vi "LvJDS2900SignalGeneratorApp.vi"() -> ()   [LabVIEW 2014]
uses:
  <vilib>/Utility/sysdir.llb/System Directory Type.ctl
  <vilib>/Utility/miscctls.llb/LVPointTypeDef.ctl
  <vilib>/Utility/error.llb/DialogType.ctl
  <vilib>/Instr/_visa.llb/VISA Configure Serial Port (Serial Instr).vi
  <vilib>/regexp/Match Regular Expression.xnode
panel:
  out "title":string="LvJDS2900SignalGeneratorApp"
  in  "Phase":dbl min=0.0 max=359.9 step=0.1 format="%0.1f"
  in  "Output 2":bool caption="Output"
  in  "Output 1":bool caption="Output"
  in  "Duty 2":dbl=50.0 caption="Duty" min=0.1 max=99.9 format="%04.1f"
  in  "Offset 2":dbl caption="Offset" min=-9.9 max=9.9 format="%04.2f"
  in  "Amplitude 2":dbl=5.0 caption="Amplitude" min=0.002 max=20.0 format="%06.3f"
  in  "WaveType 2":u16(ring) caption="WaveType" items=["Sine", "Square", "Pulse", "Triangle", "PartialSine", "CMOS", "DC"]
  in  "Frequency 2":dbl=1.0 caption="Frequency" min=1.0 max=60000000.0 format="%010.2f"
  in  "Duty 1":dbl=50.0 caption="Duty" min=0.1 max=99.9 format="%04.1f"
  in  "Offset 1":dbl caption="Offset" min=-9.99 max=9.99 format="%04.2f"
  in  "Amplitude 1":dbl=5.0 caption="Amplitude" min=0.002 max=20.0 format="%06.3f"
  in  "WaveType 1":u16(ring) caption="WaveType" items=["Sine", "Square", "Pulse", "Triangle", "PartialSine", "CMOS", "DC"]
  in  "Frequency 1":dbl=1.0 caption="Frequency" min=1.0 max=60000000.0 format="%010.2f"
  in  "VISA rscname":refnum<visa-resource-name>="COM3" caption="Port"
  in  "Btn Update":bool
  out "ModelName":string
  out "SerialNumber":string
  # "Unofficial JDS-2900 LvApp"
  # "Require NI-VISA\n\nConnect to PC via USB"
  # "As soon as the data is changed it will be sent to the device."
  # "CH1"
  # "CH2"
  # "Hz"
  # "V"
  # "V"
  # "%"
  # "Hz"
  # "V"
  # "V"
  # "%"
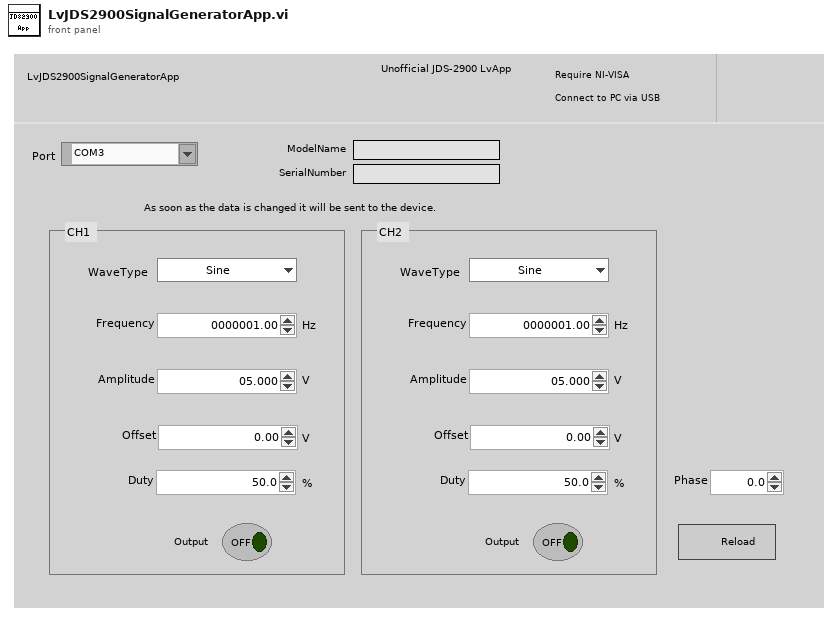
[diagram p1: front panel]
types:
  T1 = typedef "System Directory Type.ctl" = i32
  T2 = typedef "LVPointTypeDef.ctl" = cluster{"Horizontal":i16, "Vertical":i16}
  T3 = cluster{bool, "include Ctrl key?":bool, string}[]
  T4 = typedef "DialogType.ctl" = u16
  T5 = enum32{"invalid app kind", "Development System", "Run Time System", "Student Edition", "Embedded LabVIEW", "Evaluation", "Custom"}
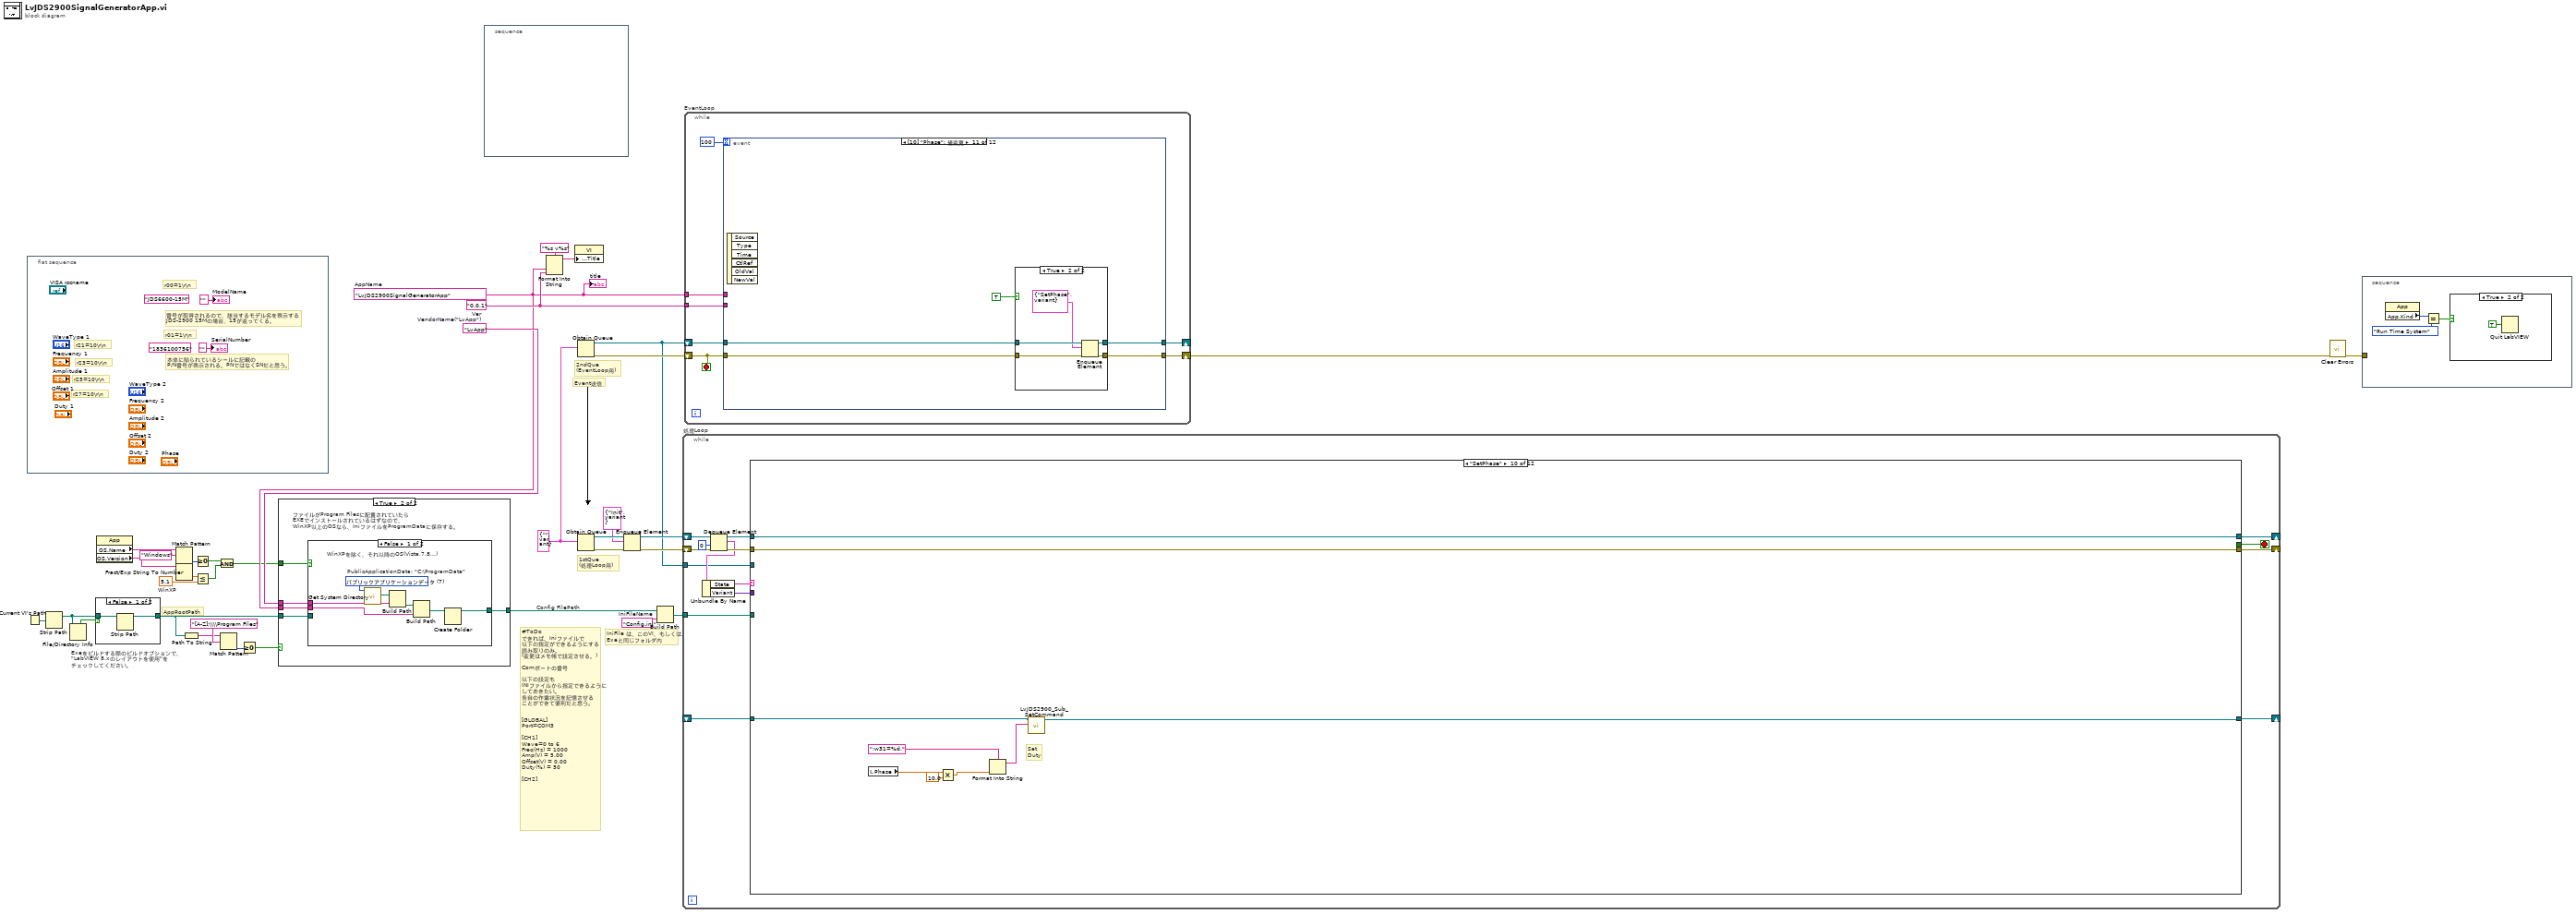
[diagram p0: block diagram]
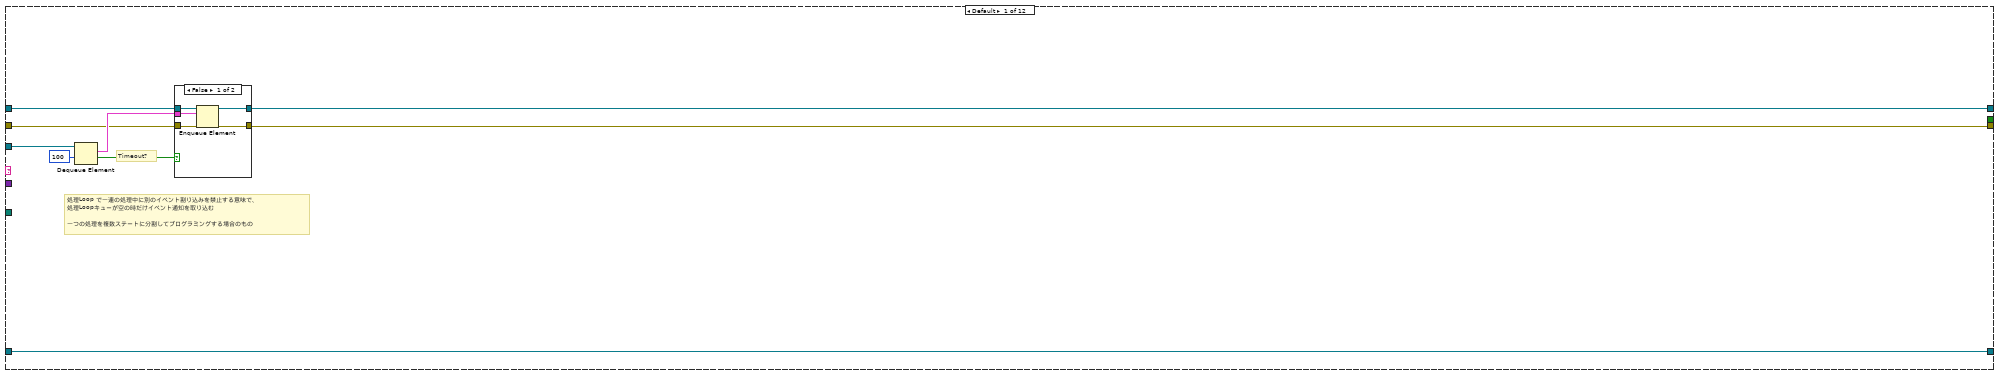
[diagram p6: hidden frame]
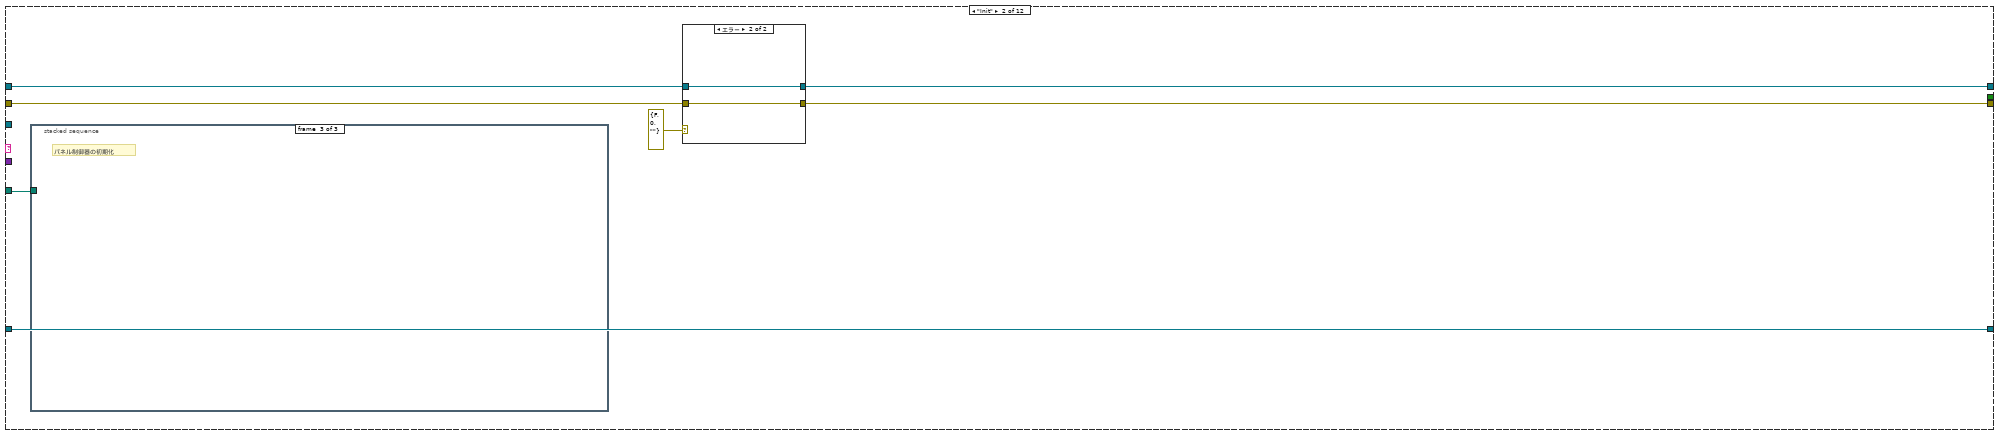
[diagram p8: hidden frame]
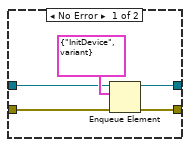
[diagram p9: hidden frame]
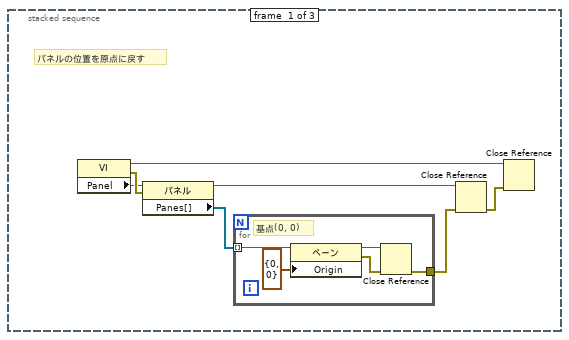
[diagram p10: hidden frame]
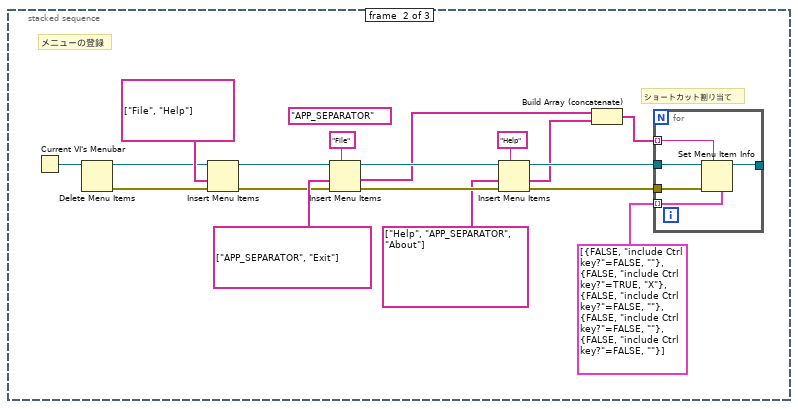
[diagram p11: hidden frame]
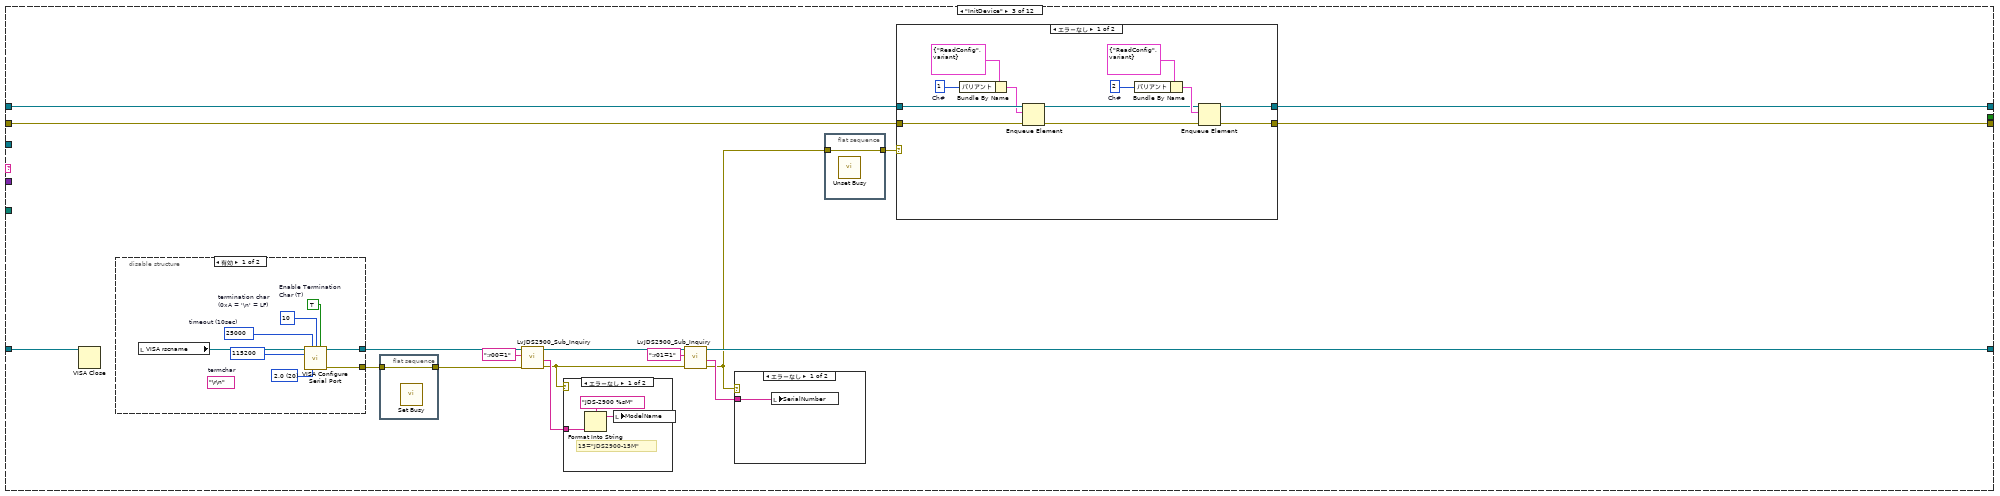
[diagram p12: hidden frame]
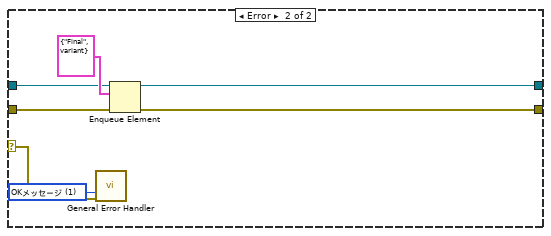
[diagram p15: hidden frame]
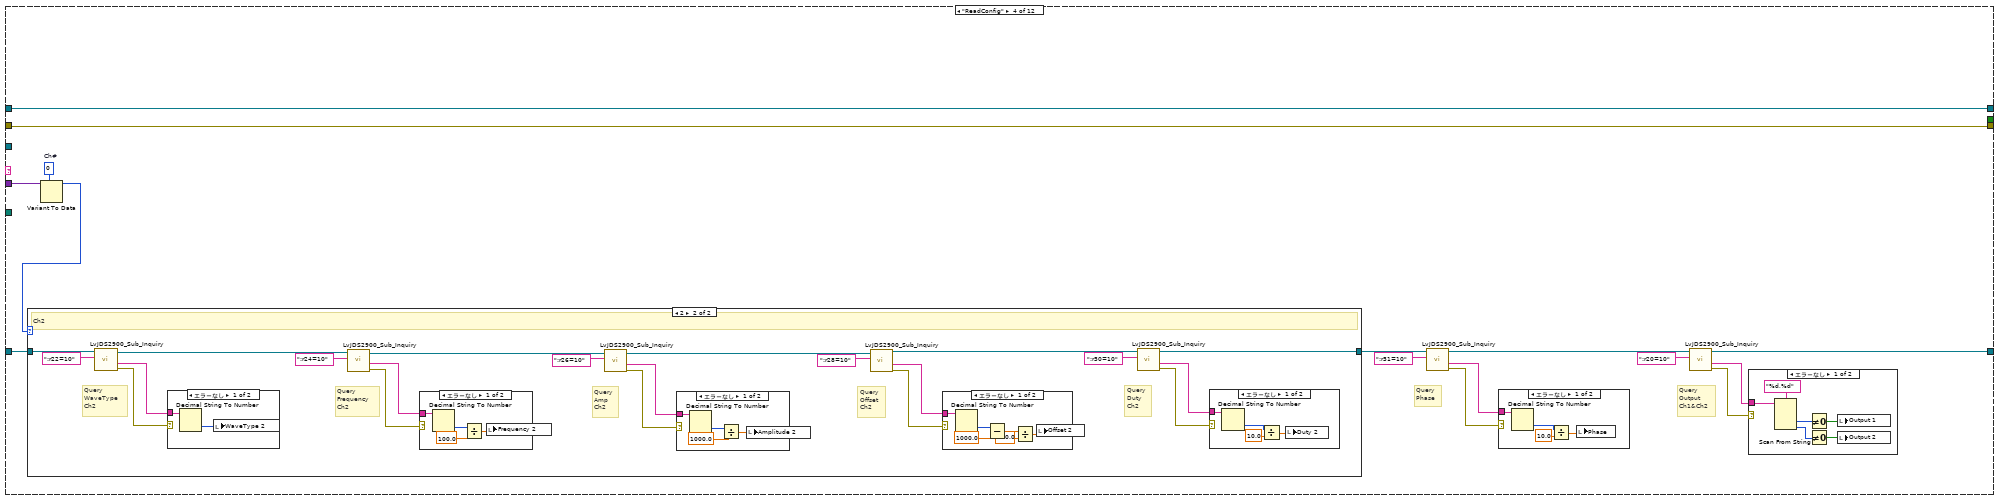
[diagram p17: hidden frame]
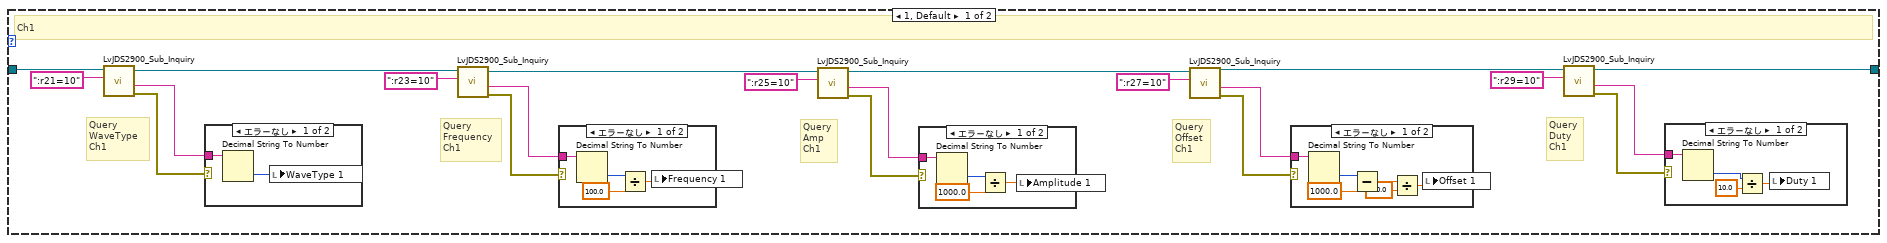
[diagram p20: hidden frame]
diagram:
  w11 = "LvApp"  # VendorName("LvApp")
  w16 = 5.1  # WinXP
  w21 = "Config.ini"  # IniFileName
  w24 = "0.0.1"  # Ver
  w10 = "LvJDS2900SignalGeneratorApp"  # AppName
  w35 = cluster{"State":string, "Variant":variant} {"State"="", "Variant"=variant}
  # "#ToDo\nできれば、Iniファイルで\n以下の指定ができるようにする\n読み取りのみ。\n(変更はメモ帳で設定させる。)\n\nComポートの番号\n\n以下の設定も\nINIファイルから指定できるように\nしておきたい。\n各自の作業状況を記憶させる\nことができて便利だと思う。\n\n\n[GLOBAL]\nPort=COM3\n\n[CH1]\nWave=0 to 6\nFreq(Hz) = 1000\nAmp(V) = 5.00\nOffset(V) = 0.00\nDuty(%) = 50\n\n[CH2]"
  # "Exeをビルドする際のビルドオプションで、\n\"LabVIEW 8.xのレイアウトを使用\"を\nチェックしてください。"
  # "Config FilePath"
  # "AppRootPath"
  # "IniFile は、このVI、もしくは、\nExeと同じフォルダ内"
  # "2ndQue\n(EventLoop用)"
  # "1stQue\n(処理Loop用)"
  # "Event送信"
  n1 = Current VI's Path() -> (path=w7:path)
  n2 = flat-sequence {
    frame #0 {
      (unwired) "1836100756" ("SerialNumber")
      (unwired) "JDS6600-15M" ("ModelName")
      # "r27=10\\r\\n"
      # "r25=10\\r\\n"
      # "r23=10\\r\\n"
      # "r21=10\\r\\n"
      # "r01=1\\r\\n"
      # "r00=1\\r\\n"
      # "本体に貼られているシールに記載の\nP/N番号が表示される。PNではなくSNだと思う。"
      # "番号が取得されるので、該当するモデル名を表示する\nJDS-2900 15Mの場合、15が返ってくる。"
      "SerialNumber" <- "" ("SerialNumber")
      "ModelName" <- "" ("ModelName")
    }
  }
  n3 = Strip Path(path=w7) -> (stripped path=w8:path)  [unwired: 1 out]
  n4 = File/Directory Info(path=w8) -> (directory=w9:bool)  [unwired: 1 in, 6 out]
  n5 = case shown="FALSE" w9 {
    tunnel: w8 -> [w39 w40]
    tunnel: [w38 w40] -> w4
    frame False {
      n6 = Strip Path(path=w39) -> (stripped path=w38:path)  [unwired: 1 out]
    }
    frame True {
    }
  }
  n7 = property class="App"() -> ("OS.Name"=w20:string, "OS.Version"=w18:string)  [unwired: 2 in, 2 out]
  n8 = Match Pattern(string=w20, regular expression="Windows" ("正規表現")) -> (offset past match=w15:i32)  [unwired: 1 in, 3 out]
  n9 = Fract/Exp String To Number(string=w18) -> (number=w17:dbl)  [unwired: 3 in, 1 out]
  n10 = Path To String(path=w4) -> (string=w3:string)
  n11 = Greater Or Equal To 0?(x=w15) -> (x >= 0?=w14:bool)
  n12 = Less Or Equal?(x=w17, y=w16) -> (x <= y?=w13:bool)
  n13 = And(x=w14, y=w13) -> (x .and. y?=w6:bool)
  n14 = Match Pattern(string=w3, regular expression="[A-Z]:\\\\Program Files" ("正規表現")) -> (offset past match=w2:i32)  [unwired: 1 in, 3 out]
  n15 = Greater Or Equal To 0?(x=w2) -> (x >= 0?=w1:bool)
  n16 = case shown="TRUE" w1 {
    tunnel: w10 -> [_ w46]
    tunnel: [w41 w44] -> w12
    tunnel: w11 -> [_ w45]
    tunnel: w6 -> [_ w43]
    tunnel: w4 -> [w41 w42]
    frame False {
      # "ファイルがProgram Filesに配置されていなかったら\n開発システムでソースから実行しているか、\nExeで適当なフォルダから実行されているので、\nIniファイルは、EXE, またはTop VI と同じ場所に保存"
    }
    frame True {
      # "ファイルがProgram Filesに配置されていたら\nEXEでインストールされているはずなので、\nWinXP以上のOSなら、IniファイルをProgramDataに保存する。"
      n17 = case shown="FALSE" w43 {
        tunnel: w46 -> [w50 _]
        tunnel: w45 -> [w48 _]
        tunnel: [w47 w54] -> w44
        tunnel: w42 -> [_ w54]
        frame False {
          w53 = T1 7 items=["ユーザホーム"=0, "ユーザデスクトップ"=1, "ユーザドキュメント"=2, "ユーザアプリケーションデータ"=3, "ユーザ設定"=4, "ユーザ一時"=5, "パブリックドキュメント"=6, "パブリックアプリケーションデータ"=7, "パブリック環境設定"=8, "パブリックキャッシュ"=13, "システムコアライブラリ"=9, "システムインストールされたライブラリ"=10, "アプリケーションファイル"=11, "ブート容量ルート"=12] ("system directory type")
          # "PublicApplicationData: \"C:\\ProgramData\""
          # "WinXPを除く、それ以降のOS(Vista,7,8,..)"
          n18 = call <vilib>:"Get System Directory.vi"("system directory type"=w53) -> ("system directory"=w52:path)  [unwired: 10 in]
          n19 = Build Path(base path=w52, name or relative path=w48) -> (appended path=w51:path)
          n20 = Build Path(base path=w51, name or relative path=w50) -> (appended path=w49:path)
          n21 = Create Folder(path (use dialog)=w49) -> (created path=w47:path)  [unwired: 2 in, 2 out]
        }
        frame True {
        }
      }
    }
  }
  n22 = stacked-sequence {
    frame #0 {
    }
  }
  n23 = Format Into String(format string="%s v%s" ("形式文字列"), w10, w24) -> (resulting string=w22:string)  [unwired: 2 in, 1 out]
  n24 = property class="VI"("Front Panel.Title"=w22) -> ()  [unwired: 2 in, 2 out]
  n25 = Obtain Queue(element data type=w35) -> (queue out=w28:refnum<queue>, error out=w34:errorcluster)  [unwired: 4 in, 1 out]
  n26 = Obtain Queue(element data type=w35) -> (queue out=w33:refnum<queue>, error out=w31:errorcluster)  [unwired: 4 in, 1 out]
  n27 = Enqueue Element(queue=w33, element=cluster{string, "バリアント":variant} {"Init", "バリアント"=variant}, error in (no error)=w31) -> (queue out=w32:refnum<queue>, error out=w30:errorcluster)  [unwired: 1 in, 1 out]
  n28 = Build Path(base path=w12, name or relative path=w21) -> (appended path=w25:path)
  n29 = while "処理Loop" {
    shift-right: [w64] -> _
    shift-left: w32 -> [w69]
    shift-right: [w63] -> _
    shift-left: w30 -> [w66]
    tunnel: w28 -> [w59]
    tunnel: w25 -> [w57]
    shift-right: [w55] -> _
    shift-left: _ -> [w56]
    stop <- w58 stop-if-true
    n30 = Dequeue Element(queue=w69, timeout in ms (-1)=0 ("タイムアウト（ms）（-1）"), error in (no error)=w66) -> (queue out=w68:refnum<queue>, element=w62:cluster{"State":string, "Variant":variant}, error out=w65:errorcluster)  [unwired: 1 out]
    n31 = Unbundle By Name(w62) -> ("State"=w61:string, "Variant"=w60:variant)
    n32 = case shown="\"SetPhase\"" w61 {
      tunnel: w68 -> [w75 w91 w150 w199 w301 w317 w333 w351 w367 w380 w390 w397]
      tunnel: w59 -> [w78 _ _ _ _ _ _ _ _ _ _ w395]
      tunnel: w65 -> [w73 w90 w149 w198 w300 w316 w332 w350 w366 w379 w389 w394]
      tunnel: [w74 w88 w147 w199 w301 w317 w333 w351 w367 w380 w390 refnum<queue> refnum ("queue out")] -> w64
      tunnel: [w72 w89 w148 w198 w300 w316 w332 w350 w366 w379 w389 w393] -> w63
      tunnel: w60 -> [_ _ _ w195 w299 w315 w331 w349 w365 _ _ _]
      tunnel: [_ _ _ _ _ _ _ _ _ _ _ TRUE] -> w58
      tunnel: w57 -> [_ w92 _ _ _ _ _ _ _ _ _ _]
      tunnel: w56 -> [w70 w87 w151 w197 w297 w313 w329 w347 w363 w378 w388 w392]
      tunnel: [w70 w87 w141 w192 w296 w312 w328 w346 w362 w377 w387 refnum<visa-resource-name> refnum ("VISA resource name out")] -> w55
      frame Default {
        # "Timeout?"
        # "処理Loop で一連の処理中に別のイベント割り込みを禁止する意味で、\n処理Loopキューが空の時だけイベント通知を取り込む\n\n一つの処理を複数ステートに分割してプログラミングする場合のもの"
        n33 = Dequeue Element(queue=w78, timeout in ms (-1)=100 ("タイムアウト（ms）（-1）")) -> (element=w76:cluster{"State":string, "Variant":variant}, timed out?=w71:bool)  [unwired: 1 in, 2 out]
        n34 = case shown="FALSE" w71 {
          tunnel: w76 -> [w83 _]
          tunnel: w75 -> [w82 w85]
          tunnel: [w81 w85] -> w74
          tunnel: w73 -> [w80 w84]
          tunnel: [w79 w84] -> w72
          frame False {
            n35 = Enqueue Element(queue=w82, element=w83, error in (no error)=w80) -> (queue out=w81:refnum<queue>, error out=w79:errorcluster)  [unwired: 1 in, 1 out]
          }
          frame True {
          }
        }
      }
      frame "Init" {
        n36 = stacked-sequence {
          tunnel: w92 -> [_ _ _]
          frame #0 {
            # "パネルの位置を原点に戻す"
            n37 = property class="VI"() -> (reference out=w103:refnum<vi>, error out=w106:errorcluster, "Panel"=w100:refnum<vi>)  [unwired: 2 in]
            n38 = property on="プロパティノード" class="パネル"(reference=w100, error in=w106) -> (reference out=w102:refnum<vi>, "Panes[]"=w101:refnum<vi>[])  [unwired: 1 out]
            n39 = for {
              tunnel: w101 -> [w111] mode=indexing
              tunnel: [w108] -> w104
              # "基点(0, 0)"
              n40 = property on="プロパティノード" class="ペーン"(reference=w111, "Origin"=T2 {"Horizontal"=0, "Vertical"=0} ("原点")) -> (reference out=w110:refnum<vi>, error out=w109:errorcluster)  [unwired: 1 in]
              n41 = Close Reference(reference=w110, error in (no error)=w109) -> (error out=w108:errorcluster)
            }
            n42 = Close Reference(reference=w102, error in (no error)=w104) -> (error out=w105:errorcluster)
            n43 = Close Reference(reference=w103, error in (no error)=w105) -> ()  [unwired: 1 out]
          }
          frame #1 {
            (unwired) "APP_SEPARATOR"
            # "ショートカット割り当て"
            # "メニューの登録"
            n44 = Current VI's Menubar() -> (w120:refnum<k9>)
            n45 = Delete Menu Items(9:w120) -> (0:w122:errorcluster, 3:w121:refnum<k9>)  [unwired: 3 in]
            n46 = Insert Menu Items(6:w122, 7:string[] ["File", "Help"] ("item tags"), 9:w121) -> (0:w126:errorcluster, 3:w125:refnum<k9>)  [unwired: 3 in, 1 out]
            n47 = Insert Menu Items(5:"File" ("menu tag"), 6:w126, 7:string[] ["APP_SEPARATOR", "Exit"] ("item tags"), 9:w125) -> (0:w129:errorcluster, 1:w115:string[], 3:w128:refnum<k9>)  [unwired: 2 in]
            n48 = Insert Menu Items(5:"Help" ("menu tag"), 6:w129, 7:string[] ["Help", "APP_SEPARATOR", "About"] ("item tags"), 9:w128) -> (0:w116:errorcluster, 1:w114:string[], 3:w117:refnum<k9>)  [unwired: 2 in]
            n49 = Build Array (concatenate)(w115, w114) -> (w112:string[])
            n50 = for {
              tunnel: w117 -> [w134]
              tunnel: w116 -> [w133]
              tunnel: [w132] -> _
              tunnel: T3 [{FALSE, "include Ctrl key?"=FALSE, ""}, {FALSE, "include Ctrl key?"=TRUE, "X"}, {FALSE, "include Ctrl key?"=FALSE, ""}, {FALSE, "include Ctrl key?"=FALSE, ""}, {FALSE, "include Ctrl key?"=FALSE, ""}] -> [w131] mode=indexing
              tunnel: w112 -> [w130] mode=indexing
              n51 = Set Menu Item Info(4:w131, 7:w130, 8:w133, 11:w134) -> (3:w132:refnum<k9>)  [unwired: 3 in, 1 out]
            }
          }
          frame #2 {
            # "パネル制御器の初期化"
          }
        }
        n52 = case shown="エラー" errorcluster {"status"=FALSE, "code"=0, "source"=""} ("error out") {
          tunnel: w91 -> [w96 w99]
          tunnel: w90 -> [w95 w98]
          tunnel: [w94 w98] -> w89
          tunnel: [w93 w99] -> w88
          frame No Error {
            n53 = Enqueue Element(queue=w96, element=cluster{string, "バリアント":variant} {"InitDevice", "バリアント"=variant}, error in (no error)=w95) -> (queue out=w93:refnum<queue>, error out=w94:errorcluster)  [unwired: 1 in, 1 out]
          }
          frame Error {
          }
        }
      }
      frame "InitDevice" {
        n54 = VISA Close(VISA resource name=w151) -> ()  [unwired: 1 in, 1 out]
        n55 = disable-structure shown="有効" {
          disable-tunnel: [w178 _] -> w146
          disable-tunnel: [w177 _] -> w136
          frame Enabled {
            (unwired) "\r\n"  # termchar
            w179 = u8 10  # termination char (0xA = '\n' = LF)
            w180 = u32 25000  # timeout (10sec)
            w181 = TRUE  # Enable Termination Char (T)
            w182 = u16 20 items=["1.0"=10, "1.5"=15, "2.0"=20] ("stop bits (10: 1 bit)")
            n56 = local read "VISA rscname"() -> (w184:refnum<visa-resource-name>)
            n57 = call-poly "VISA Configure Serial Port"("VISA resource name"=w184, "timeout (10sec)"=w180, "termination char\n(0xA = '\\n' = LF)"=w179, "Enable Termination\nChar (T)"=w181, "baud rate (9600)"=u32 115200, "stop bits (10: 1 bit)"=w182) -> ("VISA resource name out"=w178:refnum<visa-resource-name>, "error out"=w177:errorcluster)  [unwired: 8 in]
          }
          frame Disabled {
          }
        }
        n58 = flat-sequence {
          tunnel: w136 -> [w152]
          tunnel: [w152] -> w135
          frame #0 {
            n59 = call <vilib>:"Set Busy.vi"() -> ()  [unwired: 10 in, 2 out]
          }
        }
        n60 = call "LvJDS2900_Sub_Inquiry.vi"("error in (no error)"=w135, "Command"=":r00=1", "VISA rsrc"=w146) -> ("error out"=w143:errorcluster, "Response"=w144:string, "VISA rsrc out"=w142:refnum<visa-resource-name>)  [unwired: 6 in]
        n61 = case shown="エラーなし" w143 {
          tunnel: w144 -> [w156 _]
          frame No Error {
            # "15=\"JDS2900-15M\""
            n62 = Format Into String(format string="JDS-2900 %sM", w156) -> (resulting string=w154:string)  [unwired: 2 in, 1 out]
            n63 = local write "ModelName"(w154) -> ()
          }
          frame Error {
          }
        }
        n64 = call "LvJDS2900_Sub_Inquiry.vi"("error in (no error)"=w143, "Command"=":r01=1", "VISA rsrc"=w142) -> ("error out"=w138:errorcluster, "Response"=w140:string, "VISA rsrc out"=w141:refnum<visa-resource-name>)  [unwired: 6 in]
        n65 = case shown="エラーなし" w138 {
          tunnel: w140 -> [w157 _]
          frame No Error {
            n66 = local write "SerialNumber"(w157) -> ()
          }
          frame Error {
          }
        }
        n67 = flat-sequence {
          tunnel: w138 -> [w153]
          tunnel: [w153] -> w137
          frame #0 {
            n68 = call <vilib>:"Unset Busy.vi"() -> ()  [unwired: 11 in, 1 out]
          }
        }
        n69 = case shown="エラーなし" w137 {
          selector: w137 -> [_ w171]
          tunnel: w150 -> [w169 w175]
          tunnel: w149 -> [w168 w174]
          tunnel: [w158 w173] -> w148
          tunnel: [w159 w172] -> w147
          frame No Error {
            w164 = 2  # Ch#
            w165 = 1  # Ch#
            n70 = Bundle By Name(cluster=cluster{string, "バリアント":variant} {"ReadConfig", "バリアント"=variant}, "バリアント"=w165) -> (w166:cluster{string, "バリアント":variant})
            n71 = Enqueue Element(queue=w169, element=w166, error in (no error)=w168) -> (queue out=w161:refnum<queue>, error out=w160:errorcluster)  [unwired: 1 in, 1 out]
            n72 = Bundle By Name(cluster=cluster{string, "バリアント":variant} {"ReadConfig", "バリアント"=variant}, "バリアント"=w164) -> (w163:cluster{string, "バリアント":variant})
            n73 = Enqueue Element(queue=w161, element=w163, error in (no error)=w160) -> (queue out=w159:refnum<queue>, error out=w158:errorcluster)  [unwired: 1 in, 1 out]
          }
          frame Error {
            w170 = T4 1 items=["ダイアログなし", "OKメッセージ", "継続か停止メッセージ", "OKメッセージ+警告", "継続/停止+警告"] ("type of dialog (OK msg:1)")
            n74 = call <vilib>:"General Error Handler.vi"("type of dialog (OK msg:1)"=w170, "error in (no error)"=w171) -> ()  [unwired: 9 in, 5 out]
            n75 = Enqueue Element(queue=w175, element=cluster{string, "バリアント":variant} {"Final", "バリアント"=variant}, error in (no error)=w174) -> (queue out=w172:refnum<queue>, error out=w173:errorcluster)  [unwired: 1 in, 1 out]
          }
        }
      }
      frame "ReadConfig" {
        w196 = 0  # Ch#
        # "Query\nPhase"
        # "Query\nOutput\nCh1&Ch2"
        n76 = Variant To Data(type=w196, Variant=w195) -> (data=w194:i32)  [unwired: 1 in, 1 out]
        n77 = case shown="2" w194 {
          tunnel: w197 -> [w230 w271]
          tunnel: [w210 w251] -> w185
          frame 1, Default {
            # "Query\nDuty\nCh1"
            # "Query\nOffset\nCh1"
            # "Query\nAmp\nCh1"
            # "Query\nFrequency\nCh1"
            # "Query\nWaveType\nCh1"
            # "Ch1"
            n78 = call "LvJDS2900_Sub_Inquiry.vi"("Command"=":r21=10", "VISA rsrc"=w230) -> ("error out"=w229:errorcluster, "Response"=w228:string, "VISA rsrc out"=w223:refnum<visa-resource-name>)  [unwired: 7 in]
            n79 = case shown="エラーなし" w229 {
              tunnel: w228 -> [w249 _]
              frame No Error {
                n80 = Decimal String To Number(string=w249) -> (number=w250:i32)  [unwired: 2 in, 1 out]
                n81 = local write "WaveType 1"(w250) -> ()
              }
              frame Error {
              }
            }
            n82 = call "LvJDS2900_Sub_Inquiry.vi"("Command"=":r23=10", "VISA rsrc"=w223) -> ("error out"=w224:errorcluster, "Response"=w225:string, "VISA rsrc out"=w219:refnum<visa-resource-name>)  [unwired: 7 in]
            n83 = case shown="エラーなし" w224 {
              tunnel: w225 -> [w248 _]
              frame No Error {
                n84 = Decimal String To Number(string=w248) -> (number=w247:i32)  [unwired: 2 in, 1 out]
                n85 = Divide(x=w247, y=100.0) -> (x/y=w246:dbl)
                n86 = local write "Frequency 1"(w246) -> ()
              }
              frame Error {
              }
            }
            n87 = call "LvJDS2900_Sub_Inquiry.vi"("Command"=":r25=10", "VISA rsrc"=w219) -> ("error out"=w222:errorcluster, "Response"=w221:string, "VISA rsrc out"=w215:refnum<visa-resource-name>)  [unwired: 7 in]
            n88 = case shown="エラーなし" w222 {
              tunnel: w221 -> [w244 _]
              frame No Error {
                n89 = Decimal String To Number(string=w244) -> (number=w243:i32)  [unwired: 2 in, 1 out]
                n90 = Divide(x=w243, y=1000.0) -> (x/y=w241:dbl)
                n91 = local write "Amplitude 1"(w241) -> ()
              }
              frame Error {
              }
            }
            n92 = call "LvJDS2900_Sub_Inquiry.vi"("Command"=":r27=10", "VISA rsrc"=w215) -> ("error out"=w216:errorcluster, "Response"=w217:string, "VISA rsrc out"=w211:refnum<visa-resource-name>)  [unwired: 7 in]
            n93 = case shown="エラーなし" w216 {
              tunnel: w217 -> [w240 _]
              frame No Error {
                n94 = Decimal String To Number(string=w240) -> (number=w239:i32)  [unwired: 2 in, 1 out]
                n95 = Subtract(x=w239, y=1000.0) -> (x-y=w237:dbl)
                n96 = Divide(x=w237, y=100.0) -> (x/y=w236:dbl)
                n97 = local write "Offset 1"(w236) -> ()
              }
              frame Error {
              }
            }
            n98 = call "LvJDS2900_Sub_Inquiry.vi"("Command"=":r29=10", "VISA rsrc"=w211) -> ("error out"=w214:errorcluster, "Response"=w213:string, "VISA rsrc out"=w210:refnum<visa-resource-name>)  [unwired: 7 in]
            n99 = case shown="エラーなし" w214 {
              tunnel: w213 -> [w234 _]
              frame No Error {
                n100 = Decimal String To Number(string=w234) -> (number=w232:i32)  [unwired: 2 in, 1 out]
                n101 = Divide(x=w232, y=10.0) -> (x/y=w231:dbl)
                n102 = local write "Duty 1"(w231) -> ()
              }
              frame Error {
              }
            }
          }
          frame 2 {
            # "Query\nDuty\nCh2"
            # "Query\nOffset\nCh2"
            # "Query\nAmp\nCh2"
            # "Query\nFrequency\nCh2"
            # "Query\nWaveType\nCh2"
            # "Ch2"
            n103 = call "LvJDS2900_Sub_Inquiry.vi"("Command"=":r22=10", "VISA rsrc"=w271) -> ("error out"=w270:errorcluster, "Response"=w269:string, "VISA rsrc out"=w264:refnum<visa-resource-name>)  [unwired: 7 in]
            n104 = case shown="エラーなし" w270 {
              tunnel: w269 -> [w290 _]
              frame No Error {
                n105 = Decimal String To Number(string=w290) -> (number=w291:i32)  [unwired: 2 in, 1 out]
                n106 = local write "WaveType 2"(w291) -> ()
              }
              frame Error {
              }
            }
            n107 = call "LvJDS2900_Sub_Inquiry.vi"("Command"=":r24=10", "VISA rsrc"=w264) -> ("error out"=w265:errorcluster, "Response"=w266:string, "VISA rsrc out"=w260:refnum<visa-resource-name>)  [unwired: 7 in]
            n108 = case shown="エラーなし" w265 {
              tunnel: w266 -> [w289 _]
              frame No Error {
                n109 = Decimal String To Number(string=w289) -> (number=w288:i32)  [unwired: 2 in, 1 out]
                n110 = Divide(x=w288, y=100.0) -> (x/y=w287:dbl)
                n111 = local write "Frequency 2"(w287) -> ()
              }
              frame Error {
              }
            }
            n112 = call "LvJDS2900_Sub_Inquiry.vi"("Command"=":r26=10", "VISA rsrc"=w260) -> ("error out"=w263:errorcluster, "Response"=w262:string, "VISA rsrc out"=w256:refnum<visa-resource-name>)  [unwired: 7 in]
            n113 = case shown="エラーなし" w263 {
              tunnel: w262 -> [w285 _]
              frame No Error {
                n114 = Decimal String To Number(string=w285) -> (number=w284:i32)  [unwired: 2 in, 1 out]
                n115 = Divide(x=w284, y=1000.0) -> (x/y=w282:dbl)
                n116 = local write "Amplitude 2"(w282) -> ()
              }
              frame Error {
              }
            }
            n117 = call "LvJDS2900_Sub_Inquiry.vi"("Command"=":r28=10", "VISA rsrc"=w256) -> ("error out"=w257:errorcluster, "Response"=w258:string, "VISA rsrc out"=w252:refnum<visa-resource-name>)  [unwired: 7 in]
            n118 = case shown="エラーなし" w257 {
              tunnel: w258 -> [w281 _]
              frame No Error {
                n119 = Decimal String To Number(string=w281) -> (number=w280:i32)  [unwired: 2 in, 1 out]
                n120 = Subtract(x=w280, y=1000.0) -> (x-y=w278:dbl)
                n121 = Divide(x=w278, y=100.0) -> (x/y=w277:dbl)
                n122 = local write "Offset 2"(w277) -> ()
              }
              frame Error {
              }
            }
            n123 = call "LvJDS2900_Sub_Inquiry.vi"("Command"=":r30=10", "VISA rsrc"=w252) -> ("error out"=w255:errorcluster, "Response"=w254:string, "VISA rsrc out"=w251:refnum<visa-resource-name>)  [unwired: 7 in]
            n124 = case shown="エラーなし" w255 {
              tunnel: w254 -> [w275 _]
              frame No Error {
                n125 = Decimal String To Number(string=w275) -> (number=w273:i32)  [unwired: 2 in, 1 out]
                n126 = Divide(x=w273, y=10.0) -> (x/y=w272:dbl)
                n127 = local write "Duty 2"(w272) -> ()
              }
              frame Error {
              }
            }
          }
        }
        n128 = call "LvJDS2900_Sub_Inquiry.vi"("Command"=":r31=10", "VISA rsrc"=w185) -> ("error out"=w187:errorcluster, "Response"=w188:string, "VISA rsrc out"=w186:refnum<visa-resource-name>)  [unwired: 7 in]
        n129 = case shown="エラーなし" w187 {
          tunnel: w188 -> [w203 _]
          frame No Error {
            n130 = Decimal String To Number(string=w203) -> (number=w201:i32)  [unwired: 2 in, 1 out]
            n131 = Divide(x=w201, y=10.0) -> (x/y=w200:dbl)
            n132 = local write "Phase"(w200) -> ()
          }
          frame Error {
          }
        }
        n133 = call "LvJDS2900_Sub_Inquiry.vi"("Command"=":r20=10", "VISA rsrc"=w186) -> ("error out"=w190:errorcluster, "Response"=w191:string, "VISA rsrc out"=w192:refnum<visa-resource-name>)  [unwired: 7 in]
        n134 = case shown="エラーなし" w190 {
          tunnel: w191 -> [w209 _]
          frame No Error {
            n135 = Scan From String(format string="%d,%d" ("形式文字列"), input string=w209) -> (output 1=w207:i32, output 2=w205:i32)  [unwired: 4 in, 3 out]
            n136 = Not Equal To 0?(x=w207) -> (x != 0?=w206:bool)
            n137 = Not Equal To 0?(x=w205) -> (x != 0?=w204:bool)
            n138 = local write "Output 1"(w206) -> ()
            n139 = local write "Output 2"(w204) -> ()
          }
          frame Error {
          }
        }
      }
      frame "SetWaveType" {
        w298 = 0  # Ch#
        # "Set\nWaveType"
        n140 = Variant To Data(type=w298, Variant=w299) -> (data=w295:i32)  [unwired: 1 in, 1 out]
        n141 = case shown="1, デフォルト" w295 {
          tunnel: [w302 w304] -> w292
          tunnel: [":w21=%d." ":w22=%d."] -> w293
          frame 1, Default {
            n142 = local read "WaveType 1"() -> (w302:u16)
          }
          frame 2 {
            n143 = local read "WaveType 2"() -> (w304:u16)
          }
        }
        n144 = Format Into String(format string=w293, w292) -> (resulting string=w294:string)  [unwired: 2 in, 1 out]
        n145 = call "LvJDS2900_Sub_SetCommand.vi"("Command"=w294, "VISA rsrc"=w297) -> ("VISA rsrc out"=w296:refnum<visa-resource-name>)  [unwired: 8 in, 1 out]
      }
      frame "SetFrequency" {
        w314 = 0  # Ch#
        # "Set\nFrequency"
        n146 = Variant To Data(type=w314, Variant=w315) -> (data=w311:i32)  [unwired: 1 in, 1 out]
        n147 = case shown="1, デフォルト" w311 {
          tunnel: [w319 w320] -> w310
          tunnel: [":w23=%d." ":w24=%d."] -> w306
          frame 1, Default {
            n148 = local read "Frequency 1"() -> (w319:dbl)
          }
          frame 2 {
            n149 = local read "Frequency 2"() -> (w320:dbl)
          }
        }
        n150 = Multiply(x=w310, y=100.0) -> (x*y=w308:dbl)
        n151 = Format Into String(format string=w306, w308) -> (resulting string=w307:string)  [unwired: 2 in, 1 out]
        n152 = call "LvJDS2900_Sub_SetCommand.vi"("Command"=w307, "VISA rsrc"=w313) -> ("VISA rsrc out"=w312:refnum<visa-resource-name>)  [unwired: 8 in, 1 out]
      }
      frame "SetAmp" {
        w330 = 0  # Ch#
        # "Set\nAmplitude"
        n153 = Variant To Data(type=w330, Variant=w331) -> (data=w327:i32)  [unwired: 1 in, 1 out]
        n154 = case shown="2" w327 {
          tunnel: [w335 w336] -> w326
          tunnel: [":w25=%d." ":w26=%d."] -> w322
          frame 1, Default {
            n155 = local read "Amplitude 1"() -> (w335:dbl)
          }
          frame 2 {
            n156 = local read "Amplitude 2"() -> (w336:dbl)
          }
        }
        n157 = Multiply(x=w326, y=1000.0) -> (x*y=w324:dbl)
        n158 = Format Into String(format string=w322, w324) -> (resulting string=w323:string)  [unwired: 2 in, 1 out]
        n159 = call "LvJDS2900_Sub_SetCommand.vi"("Command"=w323, "VISA rsrc"=w329) -> ("VISA rsrc out"=w328:refnum<visa-resource-name>)  [unwired: 8 in, 1 out]
      }
      frame "SetOffset" {
        w348 = 0  # Ch#
        # "Set\nOffset"
        n160 = Variant To Data(type=w348, Variant=w349) -> (data=w345:i32)  [unwired: 1 in, 1 out]
        n161 = case shown="2" w345 {
          tunnel: [w352 w354] -> w344
          tunnel: [":w27=%d." ":w28=%d."] -> w340
          frame 1, Default {
            n162 = local read "Offset 1"() -> (w352:dbl)
          }
          frame 2 {
            n163 = local read "Offset 2"() -> (w354:dbl)
          }
        }
        n164 = Multiply(x=w344, y=100.0) -> (x*y=w342:dbl)
        n165 = Add(x=w342, y=1000.0) -> (x+y=w339:dbl)
        n166 = Format Into String(format string=w340, w339) -> (resulting string=w341:string)  [unwired: 2 in, 1 out]
        n167 = call "LvJDS2900_Sub_SetCommand.vi"("Command"=w341, "VISA rsrc"=w347) -> ("VISA rsrc out"=w346:refnum<visa-resource-name>)  [unwired: 8 in, 1 out]
      }
      frame "SetDuty" {
        w364 = 0  # Ch#
        # "Set\nDuty"
        n168 = Variant To Data(type=w364, Variant=w365) -> (data=w361:i32)  [unwired: 1 in, 1 out]
        n169 = case shown="2" w361 {
          tunnel: [w368 w370] -> w360
          tunnel: [":w29=%d." ":w30=%d."] -> w357
          frame 1, Default {
            n170 = local read "Duty 1"() -> (w368:dbl)
          }
          frame 2 {
            n171 = local read "Duty 2"() -> (w370:dbl)
          }
        }
        n172 = Multiply(x=w360, y=10.0) -> (x*y=w356:dbl)
        n173 = Format Into String(format string=w357, w356) -> (resulting string=w358:string)  [unwired: 2 in, 1 out]
        n174 = call "LvJDS2900_Sub_SetCommand.vi"("Command"=w358, "VISA rsrc"=w363) -> ("VISA rsrc out"=w362:refnum<visa-resource-name>)  [unwired: 8 in, 1 out]
      }
      frame "SetPhase" {
        # "Set\nDuty"
        n175 = local read "Phase"() -> (w376:dbl)
        n176 = Multiply(x=w376, y=10.0) -> (x*y=w372:dbl)
        n177 = Format Into String(format string=":w31=%d.", w372) -> (resulting string=w374:string)  [unwired: 2 in, 1 out]
        n178 = call "LvJDS2900_Sub_SetCommand.vi"("Command"=w374, "VISA rsrc"=w378) -> ("VISA rsrc out"=w377:refnum<visa-resource-name>)  [unwired: 8 in, 1 out]
      }
      frame "SetOutput" {
        # "Set\nOutput"
        n179 = local read "Output 1"() -> (w384:bool)
        n180 = local read "Output 2"() -> (w383:bool)
        n181 = Boolean To (0,1)(Boolean=w384) -> (0, 1=w382:i16)
        n182 = Boolean To (0,1)(Boolean=w383) -> (0, 1=w381:i16)
        n183 = Format Into String(format string=":w20=%d.%d.", w382, w381) -> (resulting string=w386:string)  [unwired: 2 in, 1 out]
        n184 = call "LvJDS2900_Sub_SetCommand.vi"("Command"=w386, "VISA rsrc"=w388) -> ("VISA rsrc out"=w387:refnum<visa-resource-name>)  [unwired: 8 in, 1 out]
      }
      frame "Final" {
        n185 = Release Queue(queue=w397, error in (no error)=w394) -> (error out=w393:errorcluster)  [unwired: 1 in, 2 out]
        n186 = Release Queue(queue=w395) -> ()  [unwired: 2 in, 3 out]
        n187 = VISA Close(VISA resource name=w392) -> ()  [unwired: 1 in, 1 out]
      }
    }
  }
  n188 = while "EventLoop" {
    shift-right: [w403] -> _
    shift-left: w28 -> [w404]
    shift-right: [w402] -> w27
    shift-left: w34 -> [w401]
    tunnel: w10 -> [w400]
    tunnel: w24 -> [w399]
    stop <- w401 stop-if-true
    n189 = event shown="[10] \"Phase\": 値変更" {
      selector: _ -> [_ _ _ _ _ _ _ _ _ _ _ _]
      dyn-events: _ -> [_ _ _ _ _ _ _ _ _ _ _ _]
      timeout: 100 -> [_ _ _ _ _ _ _ _ _ _ _ _]
      tunnel: w404 -> [w409 w415 w421 w429 w448 w466 w602 w738 w874 w1010 w1140 w1153]
      tunnel: [w406 w414 w420 w428 w449 w467 w603 w739 w875 w1011 w1141 w1152] -> w403
      tunnel: w401 -> [w408 w413 w419 w427 w447 w465 w601 w737 w873 w1009 w1139 w1150]
      tunnel: [w407 w412 w418 w426 w446 w464 w600 w736 w872 w1008 w1138 w1151] -> w402
      tunnel: w400 -> [_ _ _ w424 _ _ _ _ _ _ _ _]
      tunnel: w399 -> [_ _ _ w423 _ _ _ _ _ _ _ _]
      event Timeout {
        # "EventLoopの終了用"
        # "Que解放をチェック\n(終了?)"
        n190 = event-data() -> ()  [unwired: 1 in, 2 out]
        n191 = Get Queue Status(queue=w409, error in (no error)=w408) -> (queue out=w406:refnum<queue>, error out=w407:errorcluster)  [unwired: 1 in, 6 out]
      }
      event Application Instance Close? {
        n192 = event-data() -> ()  [unwired: 1 in, 4 out]
        n193 = Enqueue Element(queue=w415, element=cluster{string, "バリアント":variant} {"Final", "バリアント"=variant}, error in (no error)=w413) -> (queue out=w414:refnum<queue>, error out=w412:errorcluster)  [unwired: 1 in, 1 out]
        n194 = event-data("SilentShutdown"=TRUE, "Discard?"=FALSE ("破棄?")) -> ()  [unwired: 1 in, 1 out]
      }
      event Panel Close? {
        n195 = event-data() -> ()  [unwired: 1 in, 3 out]
        n196 = Enqueue Element(queue=w421, element=cluster{string, "バリアント":variant} {"Final", "バリアント"=variant}, error in (no error)=w419) -> (queue out=w420:refnum<queue>, error out=w418:errorcluster)  [unwired: 1 in, 1 out]
        n197 = event-data("Discard?"=TRUE) -> ()  [unwired: 1 in, 1 out]
      }
      event Menu Selection (User) {
        n198 = event-data() -> ("ItemPath"=w425:string)  [unwired: 1 in, 5 out]
        n199 = case shown="デフォルト" w425 {
          tunnel: w429 -> [w431 w436 w442 w444]
          tunnel: [w431 w435 w442 w444] -> w428
          tunnel: w427 -> [w430 w434 w441 w443]
          tunnel: [w430 w433 w441 w443] -> w426
          tunnel: w424 -> [_ _ w440 _]
          tunnel: w423 -> [_ _ w439 _]
          frame Default {
          }
          frame "File:Exit" {
            n200 = Enqueue Element(queue=w436, element=cluster{string, "バリアント":variant} {"Final", "バリアント"=variant}, error in (no error)=w434) -> (queue out=w435:refnum<queue>, error out=w433:errorcluster)  [unwired: 1 in, 1 out]
          }
          frame "Help:About" {
            n201 = Format Into String(format string="%s\n\nVersion : %s" ("メッセージ"), w440, w439) -> (resulting string=w437:string)  [unwired: 2 in, 1 out]
            n202 = One Button Dialog(message=w437) -> ()  [unwired: 1 in, 1 out]
          }
          frame "Help:Help" {
          }
        }
      }
      event "Btn Update": Value Change {
        n203 = event-data() -> ()  [unwired: 1 in, 6 out]
        n204 = case shown="TRUE" TRUE {
          tunnel: w448 -> [w451 w455]
          tunnel: w447 -> [w450 w454]
          tunnel: [w450 w453] -> w446
          tunnel: [w451 w452] -> w449
          frame False {
          }
          frame True {
            n205 = Enqueue Element(queue=w455, element=cluster{string, "バリアント":variant} {"ReadConfig", "バリアント"=variant}, error in (no error)=w454) -> (queue out=w452:refnum<queue>, error out=w453:errorcluster)  [unwired: 1 in, 1 out]
          }
        }
      }
      event "WaveType 1", "WaveType 2": Value Change {
        # "Ch#"
        n206 = event-data() -> ("CtlRef"=w462:refnum<vi>)  [unwired: 1 in, 5 out]
        n207 = property class="Ring （指定）"(reference=w462) -> ("Label.Text"=w460:string)  [unwired: 1 in, 2 out]
        n208 = xnode "正規表現で一致"("入力文字列"=w460, "正規表現"="([0-9])$") -> ("部分一致 1"=w459:string)  [unwired: 4 in, 5 out]
        n209 = Decimal String To Number(string=w459, default (0L)=1 ("デフォルト（0 I32）")) -> (number=w458:i32)  [unwired: 1 in, 1 out]
        n210 = case shown="TRUE" TRUE {
          tunnel: w466 -> [w585 w592]
          tunnel: w465 -> [w584 w591]
          tunnel: [w584 w590] -> w464
          tunnel: [w585 w589] -> w467
          tunnel: w458 -> [_ w586]
          frame False {
          }
          frame True {
            n211 = Bundle By Name(cluster=cluster{string, "バリアント":variant} {"SetWaveType", "バリアント"=variant}, "バリアント"=w586) -> (w587:cluster{string, "バリアント":variant})
            n212 = Enqueue Element(queue=w592, element=w587, error in (no error)=w591) -> (queue out=w589:refnum<queue>, error out=w590:errorcluster)  [unwired: 1 in, 1 out]
          }
        }
      }
      event "Frequency 1", "Frequency 2": Value Change {
        # "Ch#"
        n213 = event-data() -> ("CtlRef"=w598:refnum<vi>)  [unwired: 1 in, 5 out]
        n214 = property class="DigNum （指定）"(reference=w598) -> ("Label.Text"=w596:string)  [unwired: 1 in, 2 out]
        n215 = xnode "正規表現で一致"("入力文字列"=w596, "正規表現"="([0-9])$") -> ("部分一致 1"=w595:string)  [unwired: 4 in, 5 out]
        n216 = Decimal String To Number(string=w595, default (0L)=1 ("デフォルト（0 I32）")) -> (number=w594:i32)  [unwired: 1 in, 1 out]
        n217 = case shown="TRUE" TRUE {
          tunnel: w602 -> [w721 w728]
          tunnel: w601 -> [w720 w727]
          tunnel: [w720 w726] -> w600
          tunnel: [w721 w725] -> w603
          tunnel: w594 -> [_ w722]
          frame False {
          }
          frame True {
            n218 = Bundle By Name(cluster=cluster{string, "バリアント":variant} {"SetFrequency", "バリアント"=variant}, "バリアント"=w722) -> (w723:cluster{string, "バリアント":variant})
            n219 = Enqueue Element(queue=w728, element=w723, error in (no error)=w727) -> (queue out=w725:refnum<queue>, error out=w726:errorcluster)  [unwired: 1 in, 1 out]
          }
        }
      }
      event "Amplitude 1", "Amplitude 2": Value Change {
        # "Ch#"
        n220 = event-data() -> ("CtlRef"=w734:refnum<vi>)  [unwired: 1 in, 5 out]
        n221 = property class="DigNum （指定）"(reference=w734) -> ("Label.Text"=w732:string)  [unwired: 1 in, 2 out]
        n222 = xnode "正規表現で一致"("入力文字列"=w732, "正規表現"="([0-9])$") -> ("部分一致 1"=w731:string)  [unwired: 4 in, 5 out]
        n223 = Decimal String To Number(string=w731, default (0L)=1 ("デフォルト（0 I32）")) -> (number=w730:i32)  [unwired: 1 in, 1 out]
        n224 = case shown="TRUE" TRUE {
          tunnel: w738 -> [w857 w864]
          tunnel: w737 -> [w856 w863]
          tunnel: [w856 w862] -> w736
          tunnel: [w857 w861] -> w739
          tunnel: w730 -> [_ w858]
          frame False {
          }
          frame True {
            n225 = Bundle By Name(cluster=cluster{string, "バリアント":variant} {"SetAmp", "バリアント"=variant}, "バリアント"=w858) -> (w859:cluster{string, "バリアント":variant})
            n226 = Enqueue Element(queue=w864, element=w859, error in (no error)=w863) -> (queue out=w861:refnum<queue>, error out=w862:errorcluster)  [unwired: 1 in, 1 out]
          }
        }
      }
      event "Offset 1", "Offset 2": Value Change {
        # "Ch#"
        n227 = event-data() -> ("CtlRef"=w870:refnum<vi>)  [unwired: 1 in, 5 out]
        n228 = property class="DigNum （指定）"(reference=w870) -> ("Label.Text"=w868:string)  [unwired: 1 in, 2 out]
        n229 = xnode "正規表現で一致"("入力文字列"=w868, "正規表現"="([0-9])$") -> ("部分一致 1"=w867:string)  [unwired: 4 in, 5 out]
        n230 = Decimal String To Number(string=w867, default (0L)=1 ("デフォルト（0 I32）")) -> (number=w866:i32)  [unwired: 1 in, 1 out]
        n231 = case shown="TRUE" TRUE {
          tunnel: w874 -> [w993 w1000]
          tunnel: w873 -> [w992 w999]
          tunnel: [w992 w998] -> w872
          tunnel: [w993 w997] -> w875
          tunnel: w866 -> [_ w994]
          frame False {
          }
          frame True {
            n232 = Bundle By Name(cluster=cluster{string, "バリアント":variant} {"SetOffset", "バリアント"=variant}, "バリアント"=w994) -> (w995:cluster{string, "バリアント":variant})
            n233 = Enqueue Element(queue=w1000, element=w995, error in (no error)=w999) -> (queue out=w997:refnum<queue>, error out=w998:errorcluster)  [unwired: 1 in, 1 out]
          }
        }
      }
      event "Duty 1", "Duty 2": Value Change {
        # "Ch#"
        n234 = event-data() -> ("CtlRef"=w1006:refnum<vi>)  [unwired: 1 in, 5 out]
        n235 = property class="DigNum （指定）"(reference=w1006) -> ("Label.Text"=w1004:string)  [unwired: 1 in, 2 out]
        n236 = xnode "正規表現で一致"("入力文字列"=w1004, "正規表現"="([0-9])$") -> ("部分一致 1"=w1003:string)  [unwired: 4 in, 5 out]
        n237 = Decimal String To Number(string=w1003, default (0L)=1 ("デフォルト（0 I32）")) -> (number=w1002:i32)  [unwired: 1 in, 1 out]
        n238 = case shown="TRUE" TRUE {
          tunnel: w1010 -> [w1129 w1136]
          tunnel: w1009 -> [w1128 w1135]
          tunnel: [w1128 w1134] -> w1008
          tunnel: [w1129 w1133] -> w1011
          tunnel: w1002 -> [_ w1130]
          frame False {
          }
          frame True {
            n239 = Bundle By Name(cluster=cluster{string, "バリアント":variant} {"SetDuty", "バリアント"=variant}, "バリアント"=w1130) -> (w1131:cluster{string, "バリアント":variant})
            n240 = Enqueue Element(queue=w1136, element=w1131, error in (no error)=w1135) -> (queue out=w1133:refnum<queue>, error out=w1134:errorcluster)  [unwired: 1 in, 1 out]
          }
        }
      }
      event "Phase": Value Change {
        n241 = event-data() -> ()  [unwired: 1 in, 6 out]
        n242 = case shown="TRUE" TRUE {
          tunnel: w1140 -> [w1143 w1148]
          tunnel: w1139 -> [w1142 w1147]
          tunnel: [w1142 w1146] -> w1138
          tunnel: [w1143 w1145] -> w1141
          frame False {
          }
          frame True {
            n243 = Enqueue Element(queue=w1148, element=cluster{string, "バリアント":variant} {"SetPhase", "バリアント"=variant}, error in (no error)=w1147) -> (queue out=w1145:refnum<queue>, error out=w1146:errorcluster)  [unwired: 1 in, 1 out]
          }
        }
      }
      event "Output 1", "Output 2": Value Change {
        n244 = event-data() -> ()  [unwired: 1 in, 6 out]
        n245 = case shown="TRUE" TRUE {
          tunnel: w1153 -> [w1155 w1160]
          tunnel: w1150 -> [w1154 w1159]
          tunnel: [w1154 w1158] -> w1151
          tunnel: [w1155 w1157] -> w1152
          frame False {
          }
          frame True {
            n246 = Enqueue Element(queue=w1160, element=cluster{string, "バリアント":variant} {"SetOutput", "バリアント"=variant}, error in (no error)=w1159) -> (queue out=w1157:refnum<queue>, error out=w1158:errorcluster)  [unwired: 1 in, 1 out]
          }
        }
      }
    }
  }
  n247 = call <vilib>:"Clear Errors.vi"("error in (no error)"=w27) -> ("error out"=w26:errorcluster)  [unwired: 5 in, 1 out]
  n248 = stacked-sequence {
    tunnel: w26 -> [_]
    frame #0 {
      n249 = property class="App"() -> ("App.Kind"=w1163:T5)  [unwired: 2 in, 2 out]
      n250 = Equal?(x=w1163, y=T5."Run Time System" ("アプリケーション:種類")) -> (x = y?=w1161:bool)
      n251 = case shown="TRUE" w1161 {
        frame False {
        }
        frame True {
          n252 = Quit LabVIEW(quit? (T)=TRUE ("終了?（T）")) -> ()
        }
      }
    }
  }
  "title" <- w10
